vi "MenuToggle.vi"(1 "item tag":string, 2 "menubar":refnum<k9>) -> (0 "checked":bool)   [LabVIEW 2014]
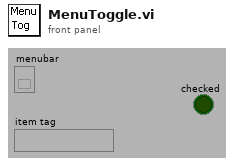
[diagram p1: front panel]
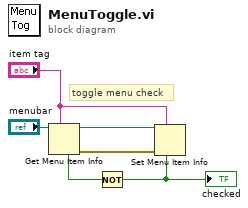
[diagram p0: block diagram]
diagram:
  # "toggle menu check"
  n1 = Get Menu Item Info(7:"item tag", 11:"menubar") -> (0:w3:errorcluster, 3:w5:refnum<k9>, 4:w4:bool)  [unwired: 1 in, 4 out]
  n2 = Not(x=w4) -> (.not. x?=w1:bool)
  "checked" <- w1
  n3 = Set Menu Item Info(6:w1, 7:"item tag", 8:w3, 11:w5) -> ()  [unwired: 3 in, 2 out]
